vi "Esercitazione 3 - Struttura IF.vi"() -> ()   [LabVIEW 2018]
panel:
  out "String 2":string
  in  "Boolean 2":bool
  out "String":string
  in  "Boolean":bool
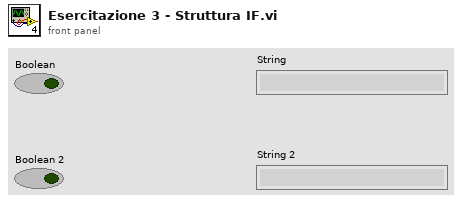
[diagram p1: front panel]
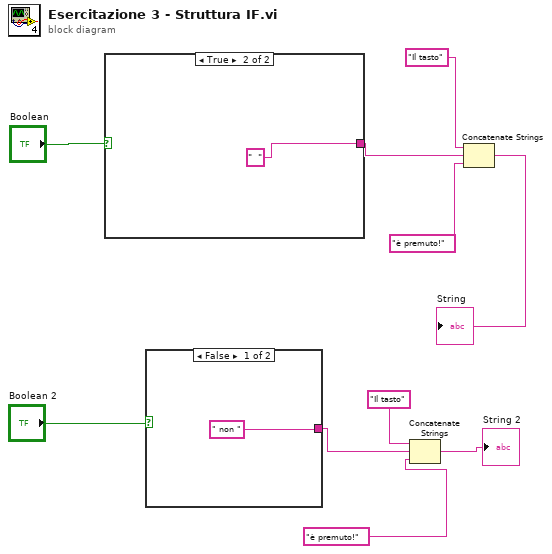
[diagram p0: block diagram]
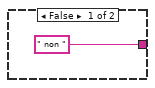
[diagram p3: hidden frame]
diagram:
  n1 = case shown="True" "Boolean" {
    tunnel: [" non " "  "] -> w7
    frame False {
    }
    frame True {
    }
  }
  n2 = case shown="False" "Boolean 2" {
    tunnel: [" non " _] -> w2
    frame False {
    }
    frame True {
    }
  }
  n3 = Concatenate Strings("Il tasto", w2, "è premuto!") -> (→"String 2":string)
  n4 = Concatenate Strings("Il tasto", w7, "è premuto!") -> (→"String":string)
